vi "ExecPratAula03.vi"() -> ()   [LabVIEW 2020]
panel:
  out "s? t:f":fxp<+/-,64,32>[](array[numeric])
  in  "Boolean":bool
  in  "Control":fxp<+/-,64,32>
  in  "Numeric 1":fxp<+/-,64,32>
  out "Slide":u8(slide) scale=0.0..200.0
  in  "Numeric 3":fxp<+/-,64,32>
  in  "Numeric 4":fxp<+/-,64,32>
  out "(i)":i32
  in  "Numeric 2":fxp<+/-,64,32>
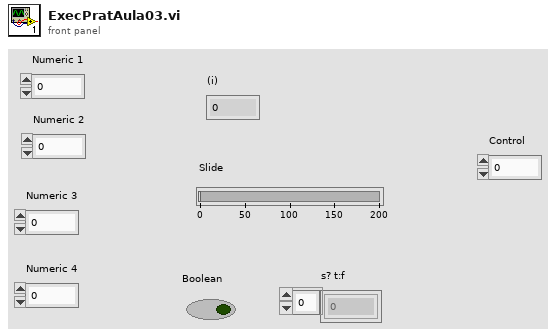
[diagram p1: front panel]
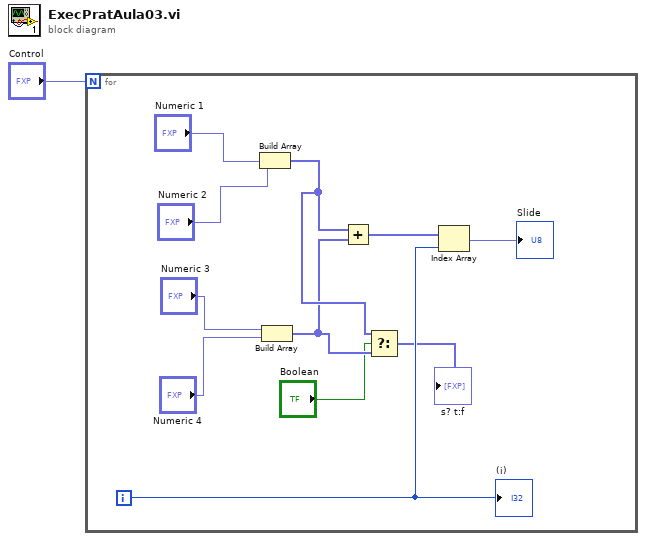
[diagram p0: block diagram]
diagram:
  n1 = for {
    N: "Control" -> [_]
    i -> [w8]
    n2 = Build Array("Numeric 1", "Numeric 2") -> (w5:fxp<+/-,64,32>[])
    n3 = Build Array("Numeric 3", "Numeric 4") -> (w3:fxp<+/-,64,32>[])
    n4 = Add(x=w5, y=w3) -> (x+y=w9:fxp<+/-,64,33>[])
    n5 = Select(t=w5, s="Boolean", f=w3) -> (s? t:f=→"s? t:f":fxp<+/-,64,32>[])
    n6 = Index Array(array=w9, index=w8) -> (element=→"Slide":fxp<+/-,64,33>)
    "(i)" <- w8
  }
